vi "Set Clock Source.vi"(5 "Device Address":T9=104 items=["0x68"=104, "0x69"=105], 9 "Clock Source":u8, 11 "error in (no error)":errorcluster) -> (15 "error out":errorcluster)   [LabVIEW 2016, in "LIFA MPU-60X0.lvlib"]
doc: "Sets the clock source.\n\n0 - Internal 8MHz oscillator\n1 - PLL with X axis gyroscope reference\n2 - PLL with Y axis gyroscope reference\n3 - PLL with Z axis gyroscope reference\n4 - PLL with external 32.768kHz reference\n5 - PLL with external 19.2MHz reference\n6 - Reserved\n7 - Stops the clock and keeps the timing generator in reset"
uses:
  LIFA MPU-60X0.lvlib
  MPU6050/DeviceAddresses.ctl
  <vilib>/myRIO/Instrument Drivers/Onboard IO/I2C/typedefs/I2C Reference.ctl
  <vilib>/myRIO/Common/Instrument Driver Framework/Utilities/typedefs/myRIO Generic Hardware Reference.ctl
  <vilib>/myRIO/Common/Instrument Driver Framework/Utilities/typedefs/Hardware Version Enum.ctl
  <vilib>/myRIO/Common/Instrument Driver Framework/Utilities/typedefs/myRIO v1.0 Reference.ctl
  <vilib>/myRIO/Common/Instrument Driver Framework/Utilities/typedefs/Generic FPGA Reference.ctl
  <vilib>/myRIO/Common/Instrument Driver Framework/myRIO v1.0/I2C/typedefs/I2C Channels Enum.ctl
  <vilib>/myRIO/Instrument Drivers/Onboard IO/I2C/typedefs/I2C Configuration.ctl
  <vilib>/myRIO/Instrument Drivers/Onboard IO/I2C/typedefs/I2C Transfer Rate.ctl
  MPU6050/RegisterAddresses.ctl
  <vilib>/Utility/error.llb/Error Cluster From Error Code.vi
  <vilib>/myRIO/Common/Instrument Driver Framework/myRIO v1.0/I2C/vis/myRIO v1.0 Write I2C.vi
  <vilib>/myRIO/Common/Instrument Driver Framework/myRIO v1.0/I2C/vis/myRIO v1.0 Read I2C.vi
  <vilib>/myRIO/Instrument Drivers/Onboard IO/I2C/I2C.lvlib
panel:
  out "I2C Ref Out":T1={"myRIO Reference"={"myRIO Model"=enum."Unknown", "myRIO Hardware Reference"={"Generic FPGA Reference"=refnum, "Allow multiple opens"=FALSE}}, "I2C Channels Enum"=enum."Not Connected", "I2C Configuration"={"I2C Transfer Rate"=enum."Fast mode (400 kbps)"}}
  in  "I2C Ref In":T1={"myRIO Reference"={"myRIO Model"=enum."Unknown", "myRIO Hardware Reference"={"Generic FPGA Reference"=refnum, "Allow multiple opens"=FALSE}}, "I2C Channels Enum"=enum."Not Connected", "I2C Configuration"={"I2C Transfer Rate"=enum."Fast mode (400 kbps)"}}
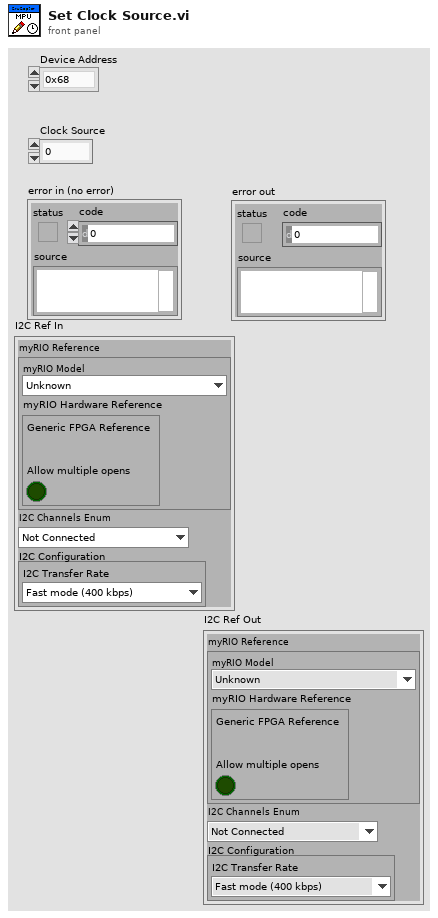
[diagram p1: front panel]
types:
  T1 = typedef "I2C.lvlib/I2C Reference.ctl" = cluster{"myRIO Reference":T2, "I2C Channels Enum":T6, "I2C Configuration":T7}
  T2 = typedef "myRIO Generic Hardware Reference.ctl" = cluster{"myRIO Model":T3, "myRIO Hardware Reference":T4}
  T3 = typedef "Hardware Version Enum.ctl" = enum16{"Unknown", "myRIO-1900", "myRIO-1950", "roboRIO", "NI ELVIS RIO CM"}
  T4 = typedef "myRIO v1.0 Reference.ctl" = cluster{"Generic FPGA Reference":T5, "Allow multiple opens":bool}
  T5 = typedef "Generic FPGA Reference.ctl" = refnum<k20>
  T6 = typedef "I2C Channels Enum.ctl" = enum16{"Not Connected", "A/I2C", "B/I2C", "I2C/I2C"}
  T7 = typedef "I2C.lvlib/I2C Configuration.ctl" = cluster{"I2C Transfer Rate":T8}
  T8 = typedef "I2C.lvlib/I2C Transfer Rate.ctl" = enum16{"Standard mode (100 kbps)", "Fast mode (400 kbps)"}
  T9 = typedef "DeviceAddresses.ctl" = u8
  T10 = typedef "RegisterAddresses.ctl" = u16
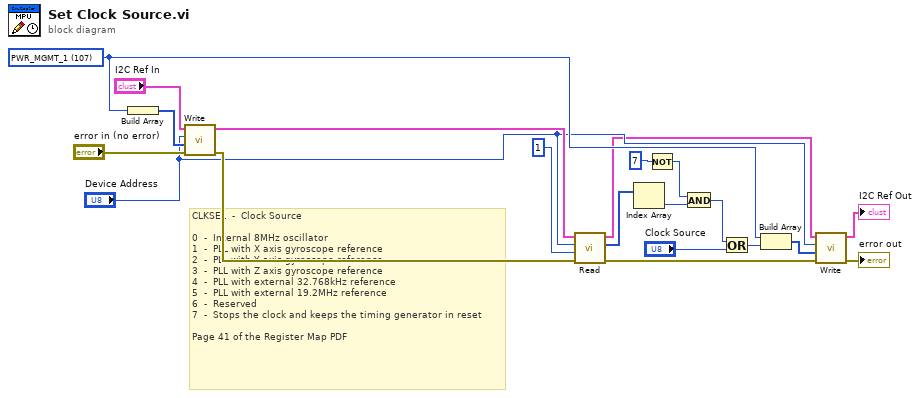
[diagram p0: block diagram]
diagram:
  w19 = T10 107 items=["SELF_TEST_X"=13, "SELF_TEST_Y"=14, "SELF_TEST_Z"=15, "SELF_TEST_A"=16, "SMPLRT_DIV"=25, "CONFIG"=26, "GYRO_CONFIG"=27, "ACCEL_CONFIG"=28, "MOT_THR"=31, "FIFO_EN"=35, "I2C_MST_CTRL"=36, "I2C_SLV0_ADDR"=37, "I2C_SLV0_REG"=38, "I2C_SLV0_CTRL"=39, "I2C_SLV1_ADDR"=40, "I2C_SLV1_REG"=41, "I2C_SLV1_CTRL"=42, "I2C_SLV2_ADDR"=43, "I2C_SLV2_REG"=44, "I2C_SLV2_CTRL"=45, "I2C_SLV3_ADDR"=46, "I2C_SLV3_REG"=47, "I2C_SLV3_CTRL"=48, "I2C_SLV4_ADDR"=49, "I2C_SLV4_REG"=50, "I2C_SLV4_DO"=51, "I2C_SLV4_CTRL"=52, "I2C_SLV4_DI"=53, "I2C_MST_STATUS"=54, "INT_PIN_CFG"=55, "INT_ENABLE"=56, "INT_STATUS"=58, "ACCEL_XOUT_H"=59, "ACCEL_XOUT_L"=60, "ACCEL_YOUT_H"=61, "ACCEL_YOUT_L"=62, "ACCEL_ZOUT_H"=63, "ACCEL_ZOUT_L"=64, "TEMP_OUT_H"=65, "TEMP_OUT_L"=66, "GYRO_XOUT_H"=67, "GYRO_XOUT_L"=68, "GYRO_YOUT_H"=69, "GYRO_YOUT_L"=70, "GYRO_ZOUT_H"=71, "GYRO_ZOUT_L"=72, "EXT_SENS_DATA_00"=73, "EXT_SENS_DATA_01"=74, "EXT_SENS_DATA_02"=75, "EXT_SENS_DATA_03"=76, "EXT_SENS_DATA_04"=77, "EXT_SENS_DATA_05"=78, "EXT_SENS_DATA_06"=79, "EXT_SENS_DATA_07"=80, "EXT_SENS_DATA_08"=81, "EXT_SENS_DATA_09"=82, "EXT_SENS_DATA_10"=83, "EXT_SENS_DATA_11"=84, "EXT_SENS_DATA_12"=85, "EXT_SENS_DATA_13"=86, "EXT_SENS_DATA_14"=87, "EXT_SENS_DATA_15"=88, "EXT_SENS_DATA_16"=89, "EXT_SENS_DATA_17"=90, "EXT_SENS_DATA_18"=91, "EXT_SENS_DATA_19"=92, "EXT_SENS_DATA_20"=93, "EXT_SENS_DATA_21"=94, "EXT_SENS_DATA_22"=95, "EXT_SENS_DATA_23"=96, "I2C_SLV0_DO"=99, "I2C_SLV1_DO"=100, "I2C_SLV2_DO"=101, "I2C_SLV3_DO"=102, "I2C_MST_DELAY_CTRL"=103, "SIGNAL_PATH_RESET"=104, "MOT_DETECT_CTRL"=105, "USER_CTRL"=106, "PWR_MGMT_1"=107, "PWR_MGMT_2"=108, "FIFO_COUNTH"=114, "FIFO_COUNTL"=115, "FIFO_R_W"=116, "WHO_AM_I"=117] ("Register Addresses")
  # "CLKSEL  -  Clock Source\n\n0  -  Internal 8MHz oscillator\n1  -  PLL with X axis gyroscope reference\n2  -  PLL with Y axis gyroscope reference\n3  -  PLL with Z axis gyroscope reference\n4  -  PLL with external 32.768kHz reference\n5  -  PLL with external 19.2MHz reference\n6  -  Reserved\n7  -  Stops the clock and keeps the timing generator in reset\n\nPage 41 of the Register Map PDF"
  n1 = Build Array(w19) -> (w12:T10[])
  n2 = call <vilib>:"Write.vi"("error in (no error)"="error in (no error)", "Bytes to Write"=w12, "Slave Address (7-bit)"="Device Address", "I2C Ref In"="I2C Ref In") -> ("error out"=w9:errorcluster, "I2C Ref Out"=w10:T1)  [unwired: 6 in]
  n3 = call <vilib>:"Read.vi"("error in (no error)"=w9, "Byte Count"=u8 1 ("Bytes To Read"), "Slave Address (7-bit)"="Device Address", "I2C Ref In"=w10) -> ("error out"=w3:errorcluster, "Bytes Read"=w8:u8[], "I2C Ref Out"=w4:T1)  [unwired: 4 in]
  n4 = Index Array(array=w8) -> (element=w18:u8)  [unwired: 1 in]
  n5 = Not(x=u8 7) -> (.not. x?=w17:u8)
  n6 = And(x=w17, y=w18) -> (x .and. y?=w15:u8)
  n7 = Or(x=w15, y="Clock Source") -> (x .or. y?=w20:u8)
  n8 = Build Array(w19, w20) -> (w6:T10[])
  n9 = call <vilib>:"Write.vi"("error in (no error)"=w3, "Bytes to Write"=w6, "Slave Address (7-bit)"="Device Address", "I2C Ref In"=w4) -> ("error out"=→"error out":errorcluster, "I2C Ref Out"=→"I2C Ref Out":T1)  [unwired: 6 in]
